vi "gratings_and_lenses.vi"() -> ()   [LabVIEW 2010]
panel:
  in  "spots":dbl[][](array[numeric])=[[0.0, 3.0, 0.0, 1.0]]
  in  "stop":bool
  # "x"
  # "y"
  # "z"
  # "I"
  # "This sample program renders a very simple version of the \"gratings and lenses\" algorithm."
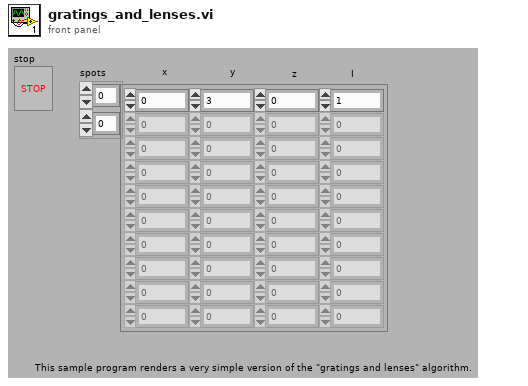
[diagram p1: front panel]
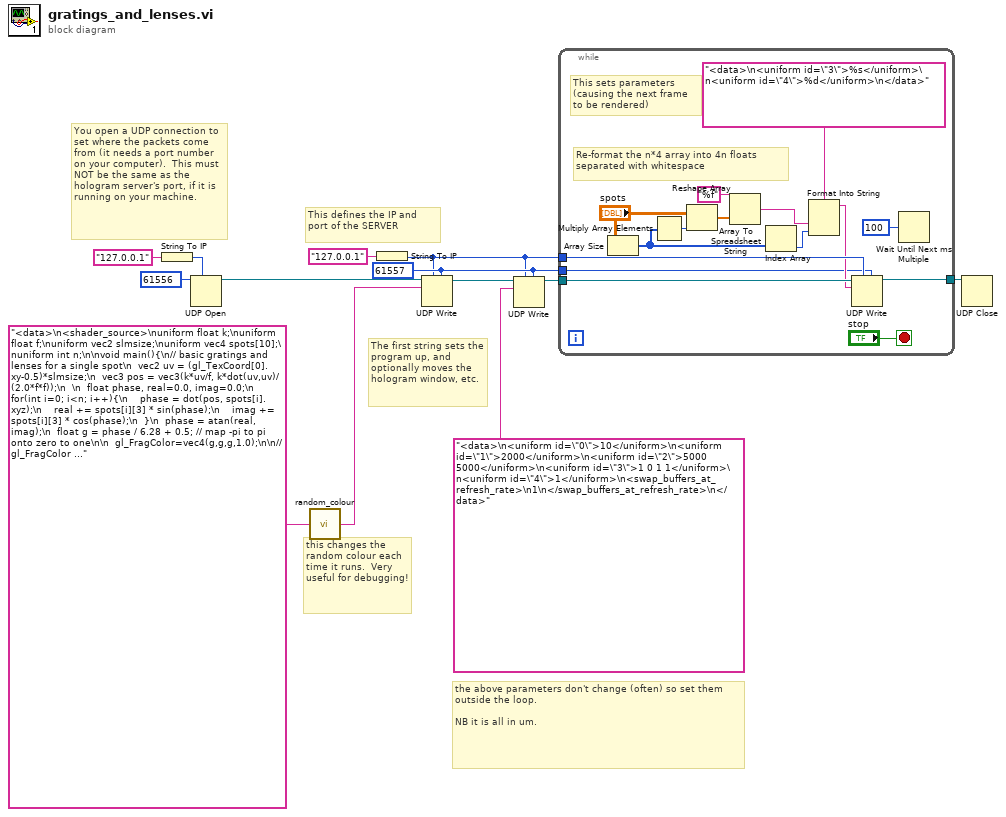
[diagram p0: block diagram]
diagram:
  w7 = u16 61557 ("port")
  # "This defines the IP and port of the SERVER"
  # "the above parameters don't change (often) so set them outside the loop.\n\nNB it is all in um."
  # "You open a UDP connection to set where the packets come from (it needs a port number on your computer).  This must NOT be the same as the hologram server's port, if it is running on your machine."
  # "The first string sets the program up, and optionally moves the hologram window, etc."
  # "this changes the random colour each time it runs.  Very useful for debugging!"
  n1 = String To IP(1:"127.0.0.1" ("name")) -> (0:w6:u32)
  n2 = UDP Open(7:w6, 11:u16 61556 ("port")) -> (port=w13:refnum<k16>)  [unwired: 3 in, 2 out]
  n3 = call "random_colour.vi"("string in"="<data>\n<shader_source>\nuniform float k;\nuniform float f;\nuniform vec2 slmsize;\nuniform vec4 spots[10];\nuniform int n;\n\nvoid main(){\n// basic gratings and lenses for a single spot\n  vec2 uv = (gl_TexCoord[0].xy-0.5)*slmsize;\n  vec3 pos = vec3(k*uv/f, k*dot(uv,uv)/(2.0*f*f));\n  \n  float phase, real=0.0, imag=0.0;\n  for(int i=0; i<n; i++){\n    phase = dot(pos, spots[i].xyz);\n    real += spots[i][3] * sin(phase);\n    imag += spots[i][3] * cos(phase);\n  }\n  phase = atan(real, imag);\n  float g = phase / 6.28 + 0.5; // map -pi to pi onto zero to one\n\n  gl_FragColor=vec4(g,g,g,1.0);\n\n//  gl_FragColor = vec4(%%randcol%%);\n}\n</shader_source>\n<window_rect>\n0 0 512 512\n</window_rect>\n</data> " ("data in")) -> ("string out, with %%randcol%% replaced with a 4-element colour"=w8:string)
  n4 = String To IP(1:"127.0.0.1" ("name")) -> (0:w1:u32)
  n5 = UDP Write(address=w1, port or service name=w7, connection ID=w13, data in=w8) -> (3:w4:refnum<k16>)  [unwired: 2 in, 1 out]
  n6 = UDP Write(address=w1, port or service name=w7, connection ID=w4, data in="<data>\n<uniform id=\"0\">10</uniform>\n<uniform id=\"1\">2000</uniform>\n<uniform id=\"2\">5000 5000</uniform>\n<uniform id=\"3\">1 0 1 1</uniform>\n<uniform id=\"4\">1</uniform>\n<swap_buffers_at_refresh_rate>\n1\n</swap_buffers_at_refresh_rate>\n</data>") -> (3:w5:refnum<k16>)  [unwired: 2 in, 1 out]
  n7 = while {
    tunnel: w5 -> [w28]
    tunnel: [w27] -> w11
    tunnel: w1 -> [w26]
    tunnel: w7 -> [w22]
    stop <- "stop" stop-if-true
    # "Re-format the n*4 array into 4n floats separated with whitespace"
    # "This sets parameters\n(causing the next frame\nto be rendered)"
    n8 = Array Size(array="spots") -> (size(s)=w21:i32[])
    n9 = Multiply Array Elements(1:w21) -> (0:w19:i32)
    n10 = Reshape Array("spots", w19) -> (w17:dbl[])
    n11 = Array To Spreadsheet String(array=w17, 3:"%f" ("format string")) -> (spreadsheet string=w16:string)  [unwired: 1 in]
    n12 = Index Array(array=w21) -> (element=w20:i32)  [unwired: 1 in]
    n13 = Format Into String(format string="<data>\n<uniform id=\"3\">%s</uniform>\n<uniform id=\"4\">%d</uniform>\n</data>" ("data in"), w16, w20) -> (resulting string=w24:string)  [unwired: 2 in, 1 out]
    n14 = UDP Write(address=w26, port or service name=w22, connection ID=w28, data in=w24) -> (3:w27:refnum<k16>)  [unwired: 2 in, 1 out]
    n15 = Wait Until Next ms Multiple(millisecond multiple=u32 100) -> ()  [unwired: 1 out]
  }
  n16 = UDP Close(connection ID=w11) -> ()  [unwired: 1 in, 2 out]
